vi "Remote Connect.vi"(2 "Error In":errorcluster, 3 "IP Address":string) -> (0 "Error Out":errorcluster, 1 "TCP":bool)   [LabVIEW 2018]
uses:
  Type Defs/Global Action.ctl
  Type Defs/RT Command.ctl
  FGVs/Global Variables.vi
  <vilib>/Utility/error.llb/Error Cluster From Error Code.vi
  <vilib>/Utility/config.llb/Write Key (String).vi
  <vilib>/ErrorRing/Error Ring.xnode
  <vilib>/Utility/config.llb/NI_LVConfig.lvlib
panel:
  out "Info":string
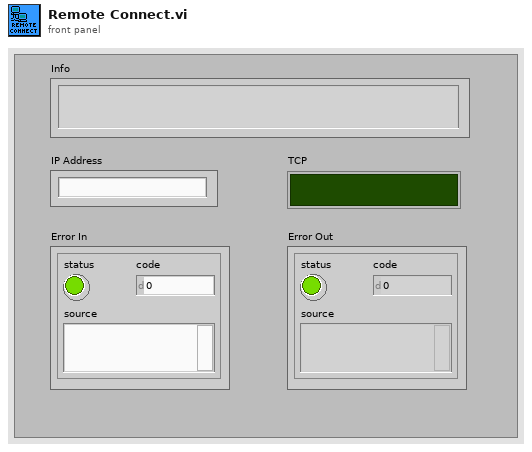
[diagram p1: front panel]
types:
  T1 = typedef "Global Action.ctl" = enum16{"Write", "Read"}
  T2 = typedef "Global Configrations.ctl" = cluster{"Model Name":enum16{"QSight 110", "QSight 120", "QSight 210", "QSight 220", "QSight 410", "QSight 420", "IONICS 3Q 110", "IONICS 3Q 120", "IONICS 3Q 210", "IONICS 3Q 220", "IONICS 3Q 310", "IONICS 3Q 320", "Simulation (Single Source)", "Simulation (Dual Source)"}, "RunType":u16, "Acquisition State":enum16{"Ready", "Busy", "Waiting"}, "InstrState":enum16{"Initializing", "Mass Spectrometer is Off", "Starting Up", "Turning Power Off", "Going to Standby", "Roughing Pump Ready", "Turning Turbo Off", "Turbo Startup", "Turbopump Ready", "Checking Vacuum", "Going to Ready", "Ready", "Running", "Source Standby", "Lost Communication", "Shutting Down", "Fault", "24V Standby", "Go to 24V Standby", "Turbopump Ready-Waiting"}, "Run Mode":enum16{"MRM (Q1/Q2)", "Q1 Scan", "Q1 SRM", "Q2 Scan", "Q2 SRM", "Product Scan", "Precursor Scan", "Neutral Loss", "Neutral Gain"}, "Configration":T3, "TCP ID":refnum<k5>, "DT":bool, "Dead Time (nS)":i32, "Single Source":bool, "ADC Tables":T5[], "FW Udate":bool, "Simulator":bool}
  T3 = typedef "Configration.ctl" = cluster{"Table":T4[], "Instrument":string[]}
  T4 = typedef "_RT Configuration 2.ctl" = cluster{"Name":string, "Ch#":u8, "Min":dbl, "Max":dbl, "Def+":dbl, "Def-":dbl, "Offset":dbl, "Slope":dbl, "Type":u8, "Description":string, "SettleT":dbl}
  T5 = typedef "ADC Table.ctl" = cluster{"Name":string, "Ch#":u8, "Min":dbl, "Max":dbl, "Def+":dbl, "Def-":dbl, "Offset":dbl, "Slope":dbl, "Type":u8, "Description":string, "SettleT":dbl}
  T6 = typedef "NI_LVConfig.lvlib/Config Data RefNum.ctl" = refnum<k1>
  T7 = typedef "RT Command.ctl" = enum16{"xml Start Run", "xml Start Actual Run", "xml Stop Run", "xml Runtime Update", "xml Get Status", "xml Get Table", "xml Set Table", "xml Get Configuration", "xml System Status", "xml Set LC Input Logic", "xml Get Data", "xml Get Info", "Start", "StartActualRun", "Stop", "Runtime Update", "Get Data", "Get Info", "Get Status", "Get Param", "Get Config", "Get Table", "Read ADC", "Set Oscillator", "Update Config", "Update Table", "Set All Pol", "Set Pol and DC", "Set Max Mass", "Toggle RP", "Toggle EL", "Set PIC", "Initialize Turbo", "Send Turbo Comm", "Close Turbo", "P1", "P2", "P3", "Send Serial", "Set LC Out", "Get LC In", "Read VAC", "Test Table", "Toggle Power", "Get Startup", "Set Startup", "Get ADC Table", "Set ADC Table", "Get Brief Status", "Get Detail Status", "Auxiliary Update", "Set CC Logics", "Set CC Input Logics", "Ignore Error", "invalid"}
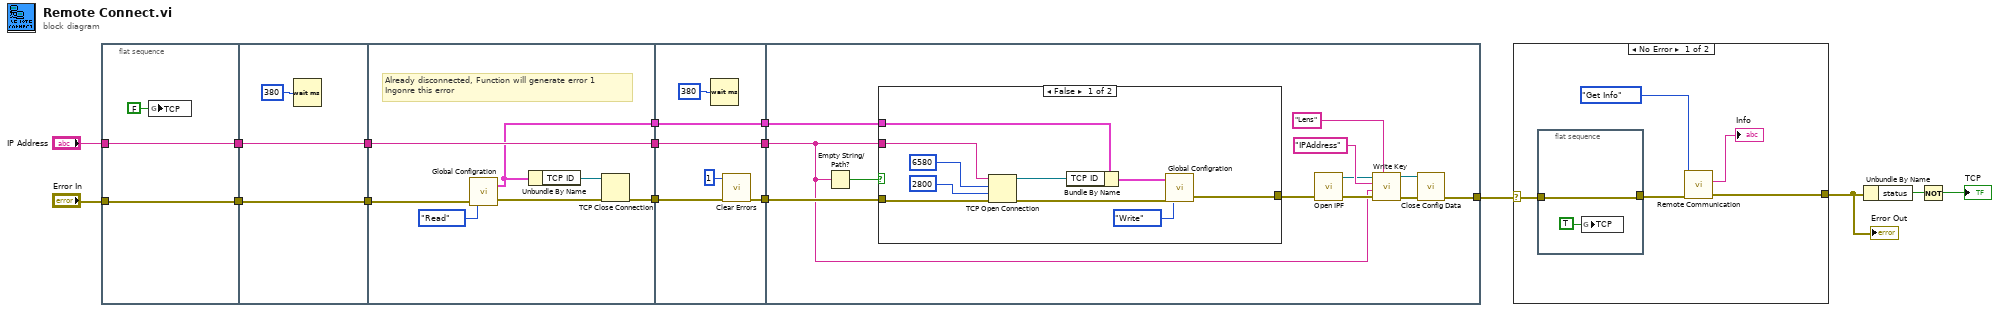
[diagram p0: block diagram]
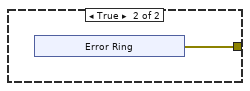
[diagram p3: hidden frame]
diagram:
  n1 = flat-sequence {
    tunnel: "Error In" -> [w18]
    tunnel: [w18] -> w9
    tunnel: [w17] -> w7
    tunnel: "IP Address" -> [w17]
    tunnel: w9 -> [w21]
    tunnel: [w21] -> w8
    tunnel: w7 -> [w20]
    tunnel: [w20] -> w4
    tunnel: [w29] -> w11
    tunnel: w8 -> [w25]
    tunnel: [w24] -> w5
    tunnel: w4 -> [w24]
    tunnel: [w23] -> w2
    tunnel: [w32] -> w12
    tunnel: w11 -> [w33]
    tunnel: w5 -> [w34]
    tunnel: [w34] -> w3
    tunnel: w2 -> [w30]
    tunnel: [w30] -> w1
    tunnel: [w38] -> w16
    tunnel: w12 -> [w46]
    tunnel: w3 -> [w37]
    tunnel: w1 -> [w36]
    frame #0 {
      n2 = global write "Global Variables.vi" "TCP"(FALSE ("TCP")) -> ()
    }
    frame #1 {
      n3 = Wait (ms)(milliseconds to wait=u32 380) -> ()  [unwired: 1 out]
    }
    frame #2 {
      # "Already disconnected, Function will generate error 1\nIngonre this error"
      n4 = call "Global Configration.vi"("Error In"=w25, "Action"=Global_Action."Read") -> ("Error Out"=w27:errorcluster, "Parameters Out"=w23:T2)  [unwired: 1 in]
      n5 = Unbundle By Name(w23) -> ("TCP ID"=w26:refnum<k5>)
      n6 = TCP Close Connection(connection ID=w26, error in (no error)=w27) -> (error out=w29:errorcluster)  [unwired: 2 out]
    }
    frame #3 {
      n7 = Wait (ms)(milliseconds to wait=u32 380) -> ()  [unwired: 1 out]
      n8 = call <vilib>:"Clear Errors.vi"("error in (no error)"=w33, "specific error code to clear (0: all)"=1) -> ("error out"=w32:errorcluster)  [unwired: 4 in, 1 out]
    }
    frame #4 {
      n9 = Empty String/Path?(string/path=w37) -> (empty?=w47:bool)
      n10 = case shown="False" w47 {
        tunnel: w46 -> [w55 _]
        tunnel: [w51 w58] -> w45
        tunnel: w37 -> [w49 _]
        tunnel: w36 -> [w48 _]
        frame False {
          n11 = TCP Open Connection(address=w49, remote port or service name=u16 6580 ("remote port"), timeout ms (60000)=2800, error in (no error)=w55) -> (connection ID=w53:refnum<k5>, error out=w54:errorcluster)  [unwired: 1 out]
          n12 = Bundle By Name(cluster=w48, "TCP ID"=w53) -> (w52:T2)
          n13 = call "Global Configration.vi"("Error In"=w54, "Action"=Global_Action."Write", "Parameters In"=w52) -> ("Error Out"=w51:errorcluster)  [unwired: 1 out]
        }
        frame True {
          n14 = xnode "Error Ring"() -> ("error out"=w58:errorcluster)
        }
      }
      n15 = call "Open IPF.vi"("Error In"=w45) -> ("Error Out"=w42:errorcluster, "IPF refnum"=w39:T6)  [unwired: 2 in, 1 out]
      n16 = call-poly <vilib>:"Write Key.vi"("section"="Lens", "error in (no error)"=w42, "value"=w37, "key"="IPAddress" ("section"), "refnum"=w39) -> ("error out"=w44:errorcluster, "refnum out"=w43:T6)  [unwired: 1 in, 4 out]
      n17 = call <vilib>:"Close Config Data.vi"("error in (no error)"=w44, "refnum"=w43) -> ("error out"=w38:errorcluster)  [unwired: 1 in, 8 out]
    }
  }
  n18 = case shown="No Error" w16 {
    selector: w16 -> [w68 w71]
    tunnel: [w64 w71] -> w15
    frame No Error {
      n19 = flat-sequence {
        tunnel: w68 -> [w69]
        tunnel: [w69] -> w67
        frame #0 {
          n20 = global write "Global Variables.vi" "TCP"(TRUE ("TCP")) -> ()
        }
      }
      n21 = call "Remote Communication.vi"("Error In"=w67, "Command"=RT_Command."Get Info") -> ("Error Out"=w64:errorcluster, "Info"=→"Info":string)  [unwired: 4 in, 2 out]
    }
    frame Error {
    }
  }
  "Error Out" <- w15
  n22 = Unbundle By Name(w15) -> ("status"=w14:bool)
  n23 = Not(x=w14) -> (.not. x?=→"TCP":bool)
